vi "NoTopBottom.vi"(2 "Value in":i32[](array[numeric]), 3 "ItemNames in":string[][](array[string])) -> (0 "Value out no change":i32[](array[numeric]), 1 "Value out":i32[](array[numeric]))   [LabVIEW 2019]
panel:
  # "This VI chops off 'top' and 'bottom' lines from the selected list if there is any."
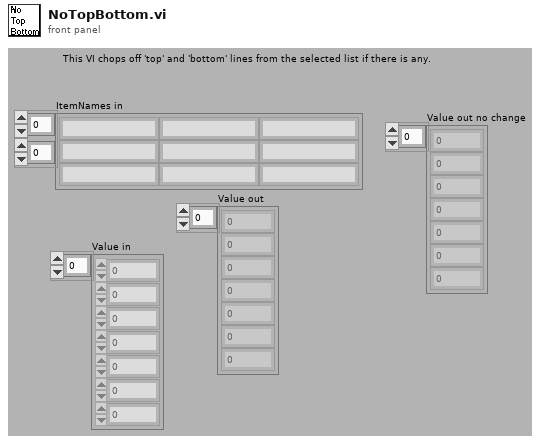
[diagram p1: front panel]
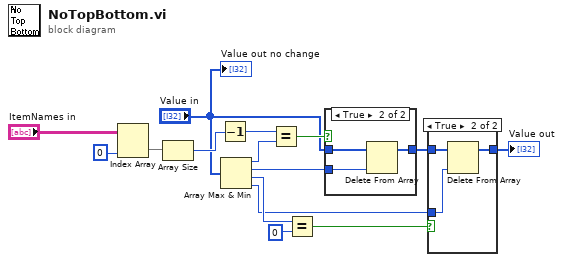
[diagram p0: block diagram]
diagram:
  n1 = Index Array(array="ItemNames in", index (col)=0 ("disabled index (col)")) -> (element=w12:string[])  [unwired: 1 in]
  n2 = Array Size(array=w12) -> (size(s)=w10:i32)
  n3 = Decrement(x=w10) -> (x-1=w14:i32)
  n4 = Array Max & Min(array="Value in") -> (max value=w15:i32, max index (indices)=w7:i32, min value=w6:i32, min index (indices)=w1:i32)
  n5 = Equal?(x=w14, y=w15) -> (x = y?=w9:bool)
  n6 = Equal?(x=w6, y=0) -> (x = y?=w4:bool)
  n7 = case shown="True" w9 {
    tunnel: "Value in" -> [w16 w19]
    tunnel: w7 -> [_ w17]
    tunnel: [w16 w18] -> w3
    frame False {
    }
    frame True {
      n8 = Delete From Array(array=w19, index=w17) -> (array with subset deleted=w18:i32[])  [unwired: 1 in, 1 out]
    }
  }
  n9 = case shown="True" w4 {
    tunnel: w3 -> [w20 w23]
    tunnel: [w20 w22] -> w2
    tunnel: w1 -> [_ w21]
    frame False {
    }
    frame True {
      n10 = Delete From Array(array=w23, index=w21) -> (array with subset deleted=w22:i32[])  [unwired: 1 in, 1 out]
    }
  }
  "Value out" <- w2
  "Value out no change" <- "Value in"
